vi "WPI_DashboardNT Log FieldName Filter.vi"(11 "Name in":string) -> (2 "Success":bool, 3 "Name out":string)   [LabVIEW 2017]
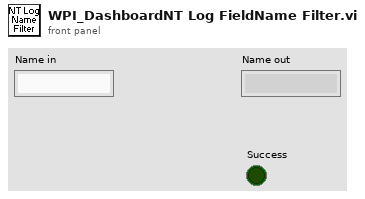
[diagram p1: front panel]
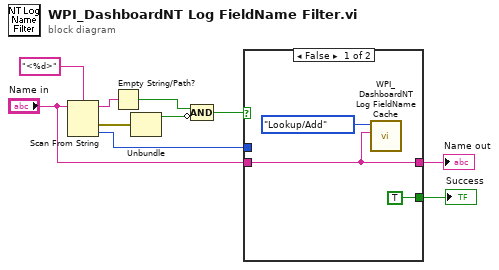
[diagram p0: block diagram]
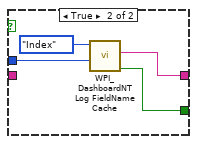
[diagram p2: hidden frame]
diagram:
  n1 = Scan From String(format string="<%d>", input string="Name in") -> (remaining string=w8:string, error out=w9:errorcluster, output 1=w4:i32)  [unwired: 3 in, 1 out]
  n2 = Empty String/Path?(string/path=w8) -> (empty?=w7:bool)
  n3 = Unbundle(w9) -> ("status"=w6:bool)  [unwired: 2 out]
  n4 = Compound Arithmetic op=AND(w7, invert w6) -> (w5:bool)
  n5 = case shown="False" w5 {
    tunnel: w4 -> [_ w17]
    tunnel: "Name in" -> [w11 _]
    tunnel: [w11 w16] -> w2
    tunnel: [TRUE w14] -> w1
    frame False {
      n6 = call <vilib>:"WPI_DashboardNT Log FieldName Cache.vi"("Name"=w11, "Operation"=enum16{"Lookup/Add", "Index"}."Lookup/Add") -> ()  [unwired: 7 in, 3 out]
    }
    frame True {
      n7 = call <vilib>:"WPI_DashboardNT Log FieldName Cache.vi"("Index"=w17, "Operation"=enum16{"Lookup/Add", "Index"}."Index") -> ("New/Valid"=w14:bool, "Name out"=w16:string)  [unwired: 7 in, 1 out]
    }
  }
  "Name out" <- w2
  "Success" <- w1
